vi "f_8_Tdoff.vi"(0 "file path (IN)":path, 1 "Project #":string, 2 "Request #":string, 3 "TEST #":string, 5 "error in (no error)":errorcluster, 6 "VGE":dbl, 8 "VCE":dbl) -> (14 "file path (OUT)":path, 15 "Tdoff (ns)":dbl, 16 "DONE Tdoff":bool, 19 "error out":errorcluster)   [LabVIEW 2020]
uses:
  GlobIndSw1.vi
  <vilib>/Waveform/WDTOps.llb/WDT Waveform Duration DBL.vi
  <vilib>/Waveform/WDTOps.llb/WDT Get Waveform Subset DBL.vi
  <vilib>/measure/mamon.llb/Trigger Detection for 1 Channel.vi
  <vilib>/Analysis/NI_AALBase.lvlib
  <vilib>/measure/NI_MAPro.lvlib
panel:
  in  "Decision ?":bool
  out "Cursor a : Channel 2":dbl
  out "Cursor a : Channel 3":dbl
  out "10% Vce":dbl
  out "90% Vge":dbl
  out "Waveform Graph":waveform(dbl)[](graph)
  out "OFF Region":waveform(dbl)[](graph) caption="Tdoff (ns)"
  # "Tdoff: from 90% Vge to 10% Vce"
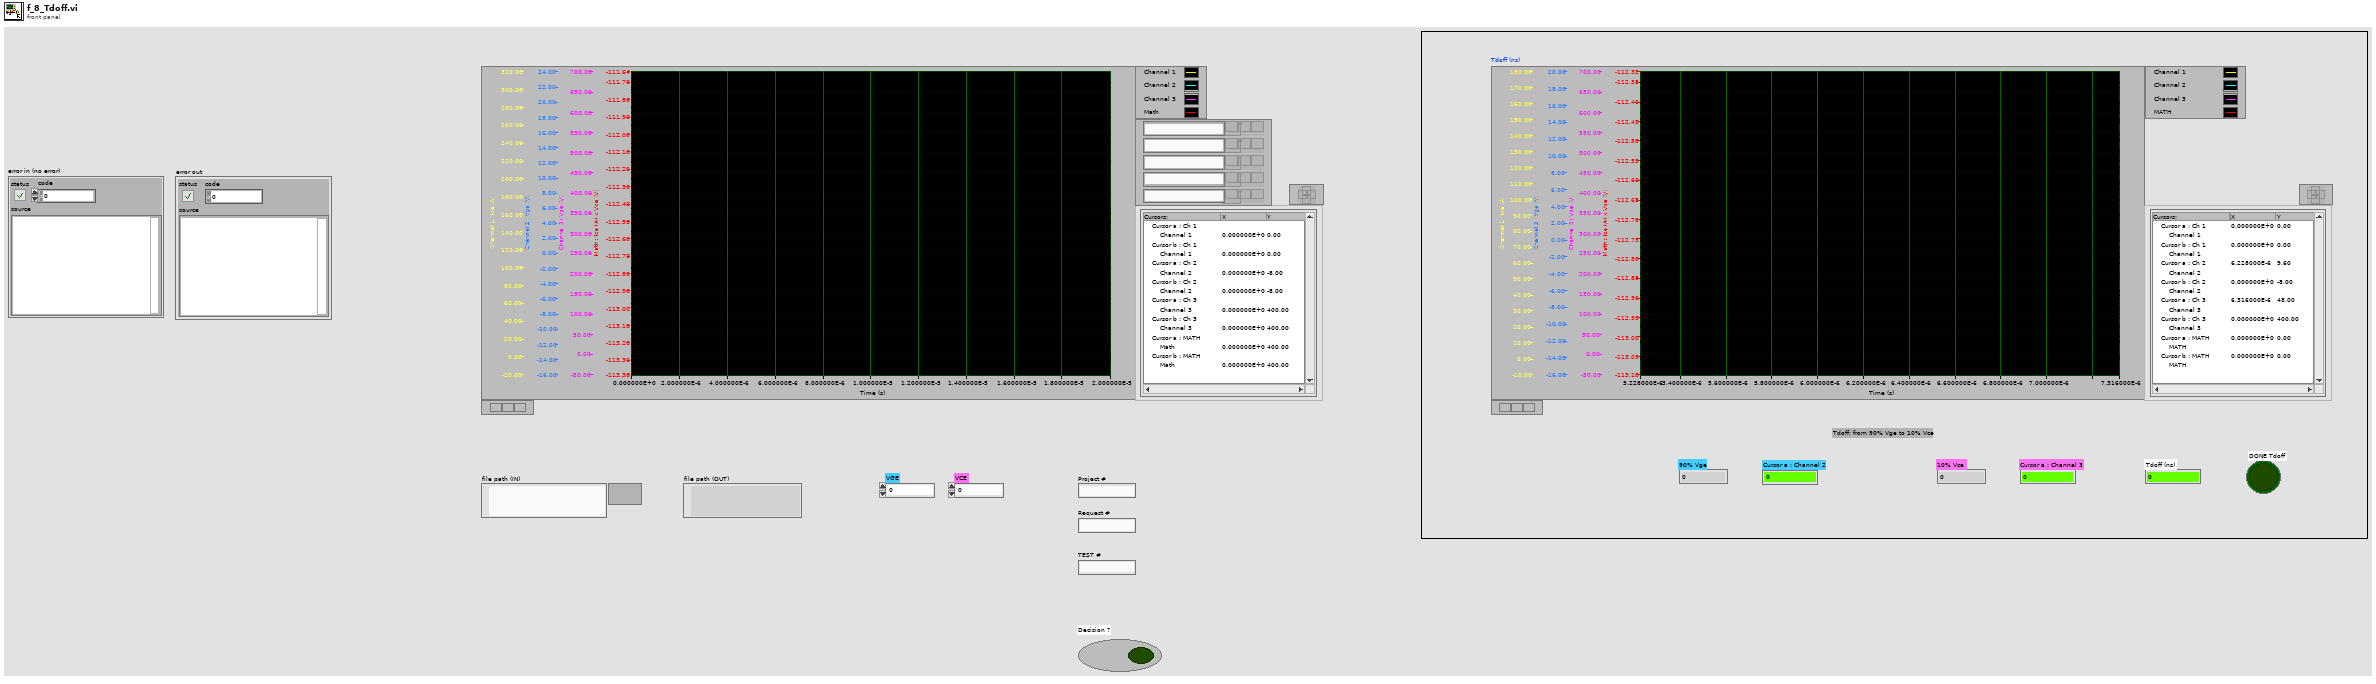
[diagram p1: front panel]
types:
  T1 = enum32{"Invalid", "Standard", "Closed", "Hidden", "Minimized", "Maximized"}
  T2 = typedef "imagedata.ctl" = cluster{"image type":i32, "image depth":i32, "image":u8[], "mask":u8[], "colors":u32[], "Rectangle":cluster{"left":i16, "top":i16, "right":i16, "bottom":i16}}
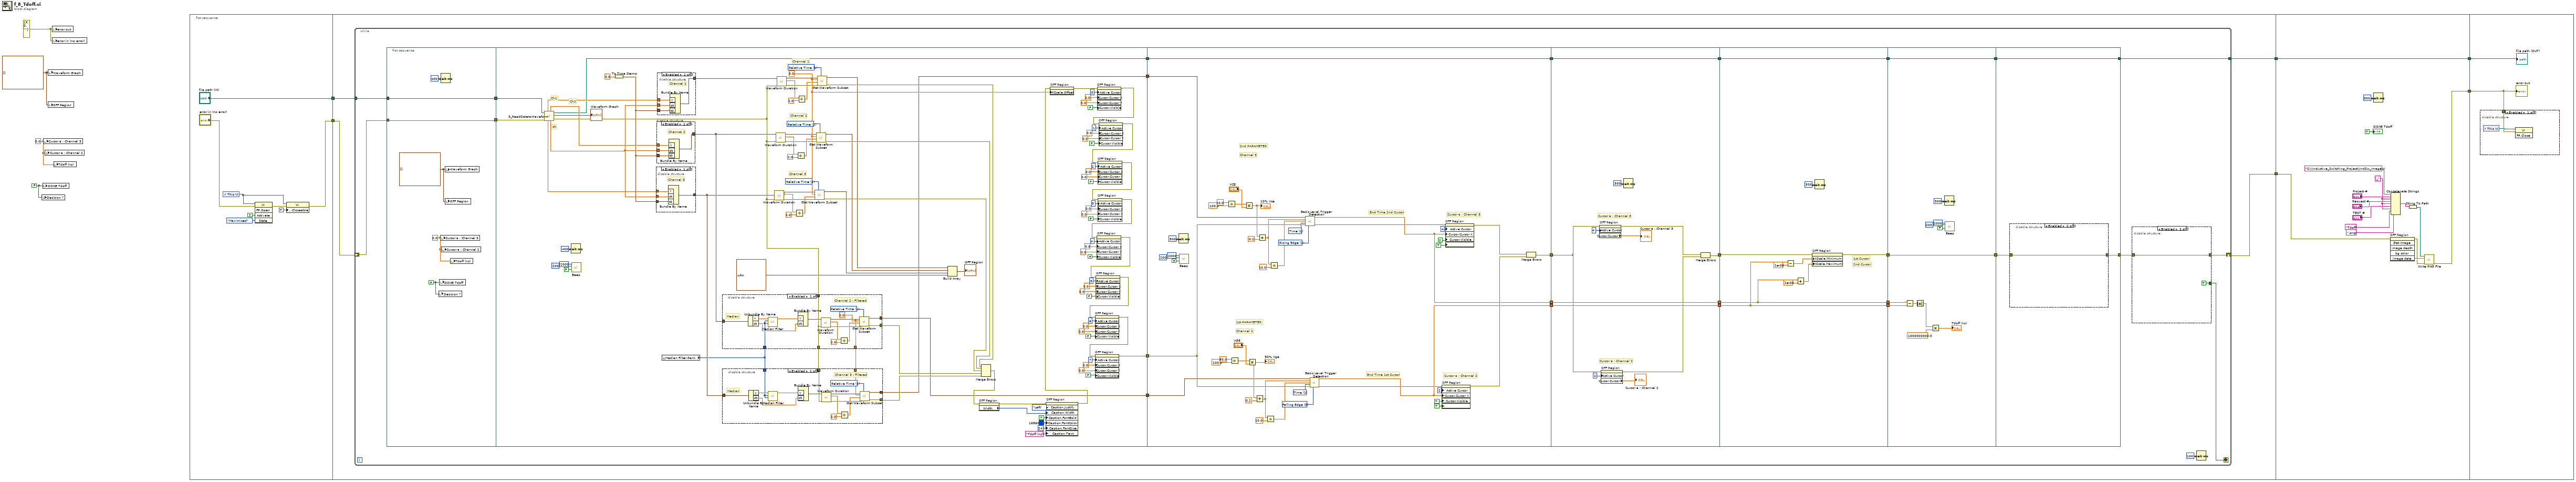
[diagram p0: block diagram]
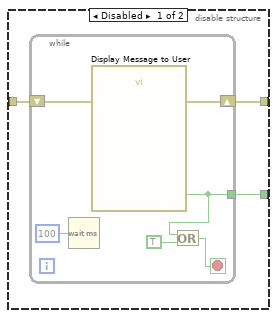
[diagram p2: hidden frame]
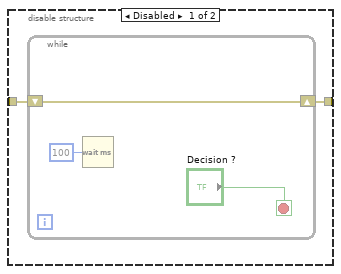
[diagram p8: hidden frame]
diagram:
  w2 = 0.0 ("Cursor a : Channel 3")
  w1 = FALSE ("DONE Tdon")
  w3 = waveform(dbl)[] [] ("Waveform Graph")
  w4 = errorcluster {"status"=FALSE, "code"=0, "source"=""} ("error out")
  n1 = local write "Decision ?"(w1) -> ()
  n2 = local write "DONE Tdoff"(w1) -> ()
  n3 = local write "Cursor a : Channel 3"(w2) -> ()
  n4 = local write "Cursor a : Channel 2"(w2) -> ()
  n5 = local write "Waveform Graph"(w3) -> ()
  n6 = local write "OFF Region"(w3) -> ()
  n7 = local write "error out"(w4) -> ()
  n8 = local write "error in (no error)"(w4) -> ()
  n9 = local write "Tdoff (ns)"(w2) -> ()
  n10 = flat-sequence {
    tunnel: ["file path (IN)"] -> w10
    tunnel: [w11] -> w9
    tunnel: w10 -> [w22]
    tunnel: [w21] -> w8
    tunnel: [w20] -> w7
    tunnel: w9 -> [w19]
    tunnel: w8 -> [w302]
    tunnel: w7 -> [w301]
    tunnel: [w301] -> w6
    tunnel: [w300] -> w5
    tunnel: w6 -> [w316]
    tunnel: w5 -> [w315]
    frame #0 {
      n11 = control-ref of="This VI"() -> (w16:refnum<vi>)
      n12 = invoke class="VI" method="FP.Open"(reference=w16, error in="error in (no error)", "Activate"=TRUE ("Activate?"), "State"=T1."Maximized") -> (error out=w17:errorcluster)  [unwired: 1 in, 4 out]
      n13 = property class="VI"(reference=w16, error in=w17, "Front Panel.Closeable"=TRUE ("Front Panel Window:Closeable")) -> (error out=w11:errorcluster)  [unwired: 1 out]
    }
    frame #1 {
      n14 = while {
        shift-right: [w27] -> w21
        shift-left: w19 -> [w23]
        tunnel: w22 -> [w25]
        tunnel: [w24] -> w20
        stop <- w28 stop-if-true
        n15 = flat-sequence {
          tunnel: [w62] -> w49
          tunnel: [w63] -> w48
          tunnel: w25 -> [w63]
          tunnel: w23 -> [w62]
          tunnel: w49 -> [w168]
          tunnel: w48 -> [w162]
          tunnel: [w71] -> w47
          tunnel: [w70] -> w46
          tunnel: [w92] -> w45
          tunnel: [w82] -> w44
          tunnel: w47 -> [w223]
          tunnel: w46 -> [w230]
          tunnel: w45 -> [w222]
          tunnel: [w229] -> w43
          tunnel: [w221] -> w42
          tunnel: [w238] -> w41
          tunnel: w44 -> [w237]
          tunnel: [w237] -> w40
          tunnel: w43 -> [w267]
          tunnel: [w267] -> w39
          tunnel: w42 -> [w266]
          tunnel: [w266] -> w38
          tunnel: w41 -> [w260]
          tunnel: [w257] -> w37
          tunnel: w40 -> [w265]
          tunnel: [w265] -> w36
          tunnel: w39 -> [w269]
          tunnel: [w269] -> w35
          tunnel: w38 -> [w270]
          tunnel: [w270] -> w34
          tunnel: w37 -> [w276]
          tunnel: [w275] -> w33
          tunnel: w36 -> [w277]
          tunnel: [w277] -> w32
          tunnel: w35 -> [w288]
          tunnel: w34 -> [w287]
          tunnel: w33 -> [w279]
          tunnel: w32 -> [w282]
          tunnel: [w282] -> w31
          tunnel: [w279] -> w30
          tunnel: w31 -> [w290]
          tunnel: w30 -> [w292]
          tunnel: [w291] -> w29
          tunnel: [w290] -> w24
          frame #0 {
            w65 = 0.0 ("Cursor a : Channel 3")
            w66 = FALSE ("DONE Tdon")
            w64 = waveform(dbl)[] [] ("Waveform Graph")
            n16 = local write "Decision ?"(w66) -> ()
            n17 = local write "DONE Tdoff"(w66) -> ()
            n18 = local write "Cursor a : Channel 3"(w65) -> ()
            n19 = Wait (ms)(milliseconds to wait=u32 400) -> ()  [unwired: 1 out]
            n20 = local write "Cursor a : Channel 2"(w65) -> ()
            n21 = local write "Waveform Graph"(w64) -> ()
            n22 = local write "OFF Region"(w64) -> ()
            n23 = local write "Tdoff (ns)"(w65) -> ()
          }
          frame #1 {
            w80 = 0.0 ("start samples/time")
            w143 = u16 1 items=["Samples", "Relative Time"] ("start/duration format")
            w154 = u16 1 items=["Samples", "Relative Time"] ("start/duration format")
            w155 = u16 1 items=["Samples", "Relative Time"] ("start/duration format")
            # "Channel 1"
            # "Channel 3"
            # "Channel 2"
            # "dt"
            # "Ch2"
            # "Ch1"
            n24 = call "3_ReadDatatoWaveform.vi"("error in (no error)"=w168, "file path (IN)"=w162) -> ("error out"=w75:errorcluster, "Waveform Graph"=→"Waveform Graph":waveform(dbl)[], "file path (OUT)"=w82:path, "dt"=w163:dbl, "Ch 2 Data"=w160:dbl[], "Ch 3 Data"=w164:dbl[], "Ch 1 Data"=w161:dbl[])  [unwired: 3 in]
            n25 = Wait (ms)(milliseconds to wait=u32 400) -> ()  [unwired: 1 out]
            n26 = call <vilib>:"Beep.vi"("use system alert? (T)"=FALSE, "duration (msec)"=u32 200, "frequency (Hz)"=u32 2000) -> ()  [unwired: 9 in]
            n27 = To Time Stamp(1:0.0 ("number")) -> (0:w165:timestamp)
            n28 = disable-structure shown="Enabled" {
              disable-tunnel: w165 -> [w212 _]
              disable-tunnel: w163 -> [w211 _]
              disable-tunnel: w164 -> [w210 _]
              disable-tunnel: [w209 _] -> w76
              frame Enabled {
                # "Channel 3"
                n29 = Bundle By Name("Y"=w210, "dt"=w211, "t0"=w212) -> (w209:waveform(dbl))  [unwired: 1 in]
              }
              frame Disabled {
              }
            }
            n30 = disable-structure shown="Enabled" {
              disable-tunnel: w165 -> [w208 _]
              disable-tunnel: w163 -> [w207 _]
              disable-tunnel: w160 -> [w206 _]
              disable-tunnel: [w205 _] -> w77
              frame Enabled {
                # "Channel 2"
                n31 = Bundle By Name("Y"=w206, "dt"=w207, "t0"=w208) -> (w205:waveform(dbl))  [unwired: 1 in]
              }
              frame Disabled {
              }
            }
            n32 = disable-structure shown="Enabled" {
              disable-tunnel: w165 -> [w204 _]
              disable-tunnel: w163 -> [w203 _]
              disable-tunnel: w161 -> [w202 _]
              disable-tunnel: [w201 _] -> w142
              frame Enabled {
                # "Channel 1"
                n33 = Bundle By Name("Y"=w202, "dt"=w203, "t0"=w204) -> (w201:waveform(dbl))  [unwired: 1 in]
              }
              frame Disabled {
              }
            }
            n34 = global read "GlobIndSw1.vi" "Median Filter Rank"() -> (w68:i32)
            n35 = disable-structure shown="Enabled" {
              disable-tunnel: w77 -> [w197 _]
              disable-tunnel: w75 -> [w187 _]
              disable-tunnel: [w189 _] -> w73
              disable-tunnel: [w188 _] -> w71
              disable-tunnel: [w187 _] -> w74
              disable-tunnel: [w186 _] -> w69
              disable-tunnel: w68 -> [w185 _]
              frame Enabled {
                w186 = 0.0 ("start samples/time")
                w191 = u16 1 items=["Samples", "Relative Time"] ("start/duration format")
                # "Channel 2 - Filtered"
                # "Median"
                n36 = Unbundle By Name(w197) -> ("Y"=w200:dbl[], "dt"=w198:dbl)
                n37 = call <vilib>:"Median Filter.vi"("right rank"=w185, "left rank"=w185, "X"=w200) -> ("Filtered X"=w199:dbl[])  [unwired: 7 in, 1 out]
                n38 = Bundle By Name("Y"=w199, "dt"=w198) -> (w190:waveform(dbl))  [unwired: 1 in]
                n39 = call-poly <vilib>:"Waveform Duration.vi"("error in (no error)"=w187, "waveform in"=w190) -> ("error out"=w194:errorcluster, "duration"=w196:dbl, "waveform out"=w195:waveform(dbl))  [unwired: 7 in]
                n40 = Divide(x=w196, y=2.0) -> (x/y=w193:dbl)
                n41 = call-poly <vilib>:"Get Waveform Subset.vi"("start/duration format"=w191, "error in (no error)"=w194, "duration"=w193, "start samples/time"=w186, "waveform in"=w195) -> ("error out"=w189:errorcluster, "waveform out"=w188:waveform(dbl))  [unwired: 1 in, 2 out]
              }
              frame Disabled {
              }
            }
            n42 = disable-structure shown="Enabled" {
              disable-tunnel: w76 -> [w181 _]
              disable-tunnel: w74 -> [w173 _]
              disable-tunnel: [w172 _] -> w72
              disable-tunnel: [w171 _] -> w70
              disable-tunnel: w69 -> [w170 _]
              disable-tunnel: w68 -> [w169 _]
              frame Enabled {
                w175 = u16 1 items=["Samples", "Relative Time"] ("start/duration format")
                # "Channel 3 - Filtered"
                # "Median"
                n43 = Unbundle By Name(w181) -> ("Y"=w184:dbl[], "dt"=w182:dbl)
                n44 = call <vilib>:"Median Filter.vi"("right rank"=w169, "left rank"=w169, "X"=w184) -> ("Filtered X"=w183:dbl[])  [unwired: 7 in, 1 out]
                n45 = Bundle By Name("Y"=w183, "dt"=w182) -> (w174:waveform(dbl))  [unwired: 1 in]
                n46 = call-poly <vilib>:"Waveform Duration.vi"("error in (no error)"=w173, "waveform in"=w174) -> ("error out"=w178:errorcluster, "duration"=w180:dbl, "waveform out"=w179:waveform(dbl))  [unwired: 7 in]
                n47 = Divide(x=w180, y=2.0) -> (x/y=w177:dbl)
                n48 = call-poly <vilib>:"Get Waveform Subset.vi"("start/duration format"=w175, "error in (no error)"=w178, "duration"=w177, "start samples/time"=w170, "waveform in"=w179) -> ("error out"=w172:errorcluster, "waveform out"=w171:waveform(dbl))  [unwired: 1 in, 2 out]
              }
              frame Disabled {
              }
            }
            n49 = call-poly <vilib>:"Waveform Duration.vi"("error in (no error)"=w75, "waveform in"=w76) -> ("error out"=w148:errorcluster, "duration"=w145:dbl, "waveform out"=w147:waveform(dbl))  [unwired: 7 in]
            n50 = call-poly <vilib>:"Waveform Duration.vi"("error in (no error)"=w75, "waveform in"=w77) -> ("error out"=w149:errorcluster, "duration"=w152:dbl, "waveform out"=w150:waveform(dbl))  [unwired: 7 in]
            n51 = call-poly <vilib>:"Waveform Duration.vi"("error in (no error)"=w75, "waveform in"=w142) -> ("error out"=w159:errorcluster, "duration"=w156:dbl, "waveform out"=w158:waveform(dbl))  [unwired: 7 in]
            n52 = Divide(x=w145, y=2.0) -> (x/y=w144:dbl)
            n53 = Divide(x=w152, y=2.0) -> (x/y=w153:dbl)
            n54 = Divide(x=w156, y=2.0) -> (x/y=w140:dbl)
            n55 = call-poly <vilib>:"Get Waveform Subset.vi"("start/duration format"=w143, "error in (no error)"=w148, "duration"=w144, "start samples/time"=w80, "waveform in"=w147) -> ("error out"=w79:errorcluster, "waveform out"=w81:waveform(dbl))  [unwired: 1 in, 2 out]
            n56 = call-poly <vilib>:"Get Waveform Subset.vi"("start/duration format"=w154, "error in (no error)"=w149, "duration"=w153, "start samples/time"=w80, "waveform in"=w150) -> ("error out"=w138:errorcluster, "waveform out"=w94:waveform(dbl))  [unwired: 1 in, 2 out]
            n57 = call-poly <vilib>:"Get Waveform Subset.vi"("start/duration format"=w155, "error in (no error)"=w159, "duration"=w140, "start samples/time"=w80, "waveform in"=w158) -> ("error out"=w139:errorcluster, "waveform out"=w93:waveform(dbl))  [unwired: 1 in, 2 out]
            n58 = Build Array(w93, w94, w81, waveform(dbl) {"t0"=timestamp(0 s since 1904-01-01), "dt"=1.0, "Y"=[]} ("element")) -> (→"OFF Region":waveform(dbl)[])
            n59 = Merge Errors(w139, w138, w79, w73, w72) -> (w90:errorcluster)
            n60 = property on="OFF Region" class="WFGraph (strict)"(error in=w90) -> (error out=w89:errorcluster, "Width"=w88:u32)  [unwired: 1 in, 1 out]
            n61 = property on="OFF Region" class="WFGraph (strict)"(error in=w89, "Caption.Justify"=enum16{"Left", "Center", "Right"}."Left" ("Caption.Justification"), "Caption.Width"=w88, "Caption.FontBold"=TRUE ("Caption.Font:Bold"), "Caption.FontColor"=u32 16860 ("Caption.Font:Color"), "Caption.FontSize"=u32 24 ("Caption.Font:Size"), "Caption.Text"="Tdoff (ns)") -> (error out=w84:errorcluster)  [unwired: 1 in, 1 out]
            n62 = property on="OFF Region" class="WFGraph (strict)"(error in=w84, "XScale.Offset"=w80) -> (error out=w118:errorcluster)  [unwired: 1 in, 1 out]
            n63 = property on="OFF Region" class="WFGraph (strict)"(error in=w118, "Active Cursor"=u32 0, "Cursor.Cursor X"=0.0 ("Cursor.Cursor Position:Cursor X"), "Cursor.Cursor Y"=0.0 ("Cursor.Cursor Position:Cursor Y"), "Cursor.Visible"=FALSE) -> (error out=w117:errorcluster)  [unwired: 1 in, 1 out]
            n64 = property on="OFF Region" class="WFGraph (strict)"(error in=w117, "Active Cursor"=u32 1, "Cursor.Cursor X"=0.0 ("Cursor.Cursor Position:Cursor X"), "Cursor.Cursor Y"=0.0 ("Cursor.Cursor Position:Cursor Y"), "Cursor.Visible"=FALSE) -> (error out=w116:errorcluster)  [unwired: 1 in, 1 out]
            n65 = property on="OFF Region" class="WFGraph (strict)"(error in=w116, "Active Cursor"=u32 2, "Cursor.Cursor X"=0.0 ("Cursor.Cursor Position:Cursor X"), "Cursor.Cursor Y"=0.0 ("Cursor.Cursor Position:Cursor Y"), "Cursor.Visible"=FALSE) -> (error out=w115:errorcluster)  [unwired: 1 in, 1 out]
            n66 = property on="OFF Region" class="WFGraph (strict)"(error in=w115, "Active Cursor"=u32 3, "Cursor.Cursor X"=0.0 ("Cursor.Cursor Position:Cursor X"), "Cursor.Cursor Y"=0.0 ("Cursor.Cursor Position:Cursor Y"), "Cursor.Visible"=FALSE) -> (error out=w98:errorcluster)  [unwired: 1 in, 1 out]
            n67 = property on="OFF Region" class="WFGraph (strict)"(error in=w98, "Active Cursor"=u32 4, "Cursor.Cursor X"=0.0 ("Cursor.Cursor Position:Cursor X"), "Cursor.Cursor Y"=0.0 ("Cursor.Cursor Position:Cursor Y"), "Cursor.Visible"=FALSE) -> (error out=w97:errorcluster)  [unwired: 1 in, 1 out]
            n68 = property on="OFF Region" class="WFGraph (strict)"(error in=w97, "Active Cursor"=u32 5, "Cursor.Cursor X"=0.0 ("Cursor.Cursor Position:Cursor X"), "Cursor.Cursor Y"=0.0 ("Cursor.Cursor Position:Cursor Y"), "Cursor.Visible"=FALSE) -> (error out=w96:errorcluster)  [unwired: 1 in, 1 out]
            n69 = property on="OFF Region" class="WFGraph (strict)"(error in=w96, "Active Cursor"=u32 6, "Cursor.Cursor X"=0.0 ("Cursor.Cursor Position:Cursor X"), "Cursor.Cursor Y"=0.0 ("Cursor.Cursor Position:Cursor Y"), "Cursor.Visible"=FALSE) -> (error out=w95:errorcluster)  [unwired: 1 in, 1 out]
            n70 = property on="OFF Region" class="WFGraph (strict)"(error in=w95, "Active Cursor"=u32 7, "Cursor.Cursor X"=0.0 ("Cursor.Cursor Position:Cursor X"), "Cursor.Cursor Y"=0.0 ("Cursor.Cursor Position:Cursor Y"), "Cursor.Visible"=FALSE) -> (error out=w92:errorcluster)  [unwired: 1 in, 1 out]
          }
          frame #2 {
            w226 = u16 0 items=["Falling Edge", "Rising Edge"] ("trigger slope")
            w227 = u16 1 items=["Index", "Time"] ("location mode")
            w233 = u16 1 items=["Falling Edge", "Rising Edge"] ("trigger slope")
            w234 = u16 1 items=["Index", "Time"] ("location mode")
            # "Cursor a : Channel 2"
            # "Cursor a : Channel 3"
            # "End Time 2nd Cursor"
            # "End Time 1st Cursor"
            # "2nd PARAMETER"
            # "Channel 3"
            # "1st PARAMETER"
            # "Channel 2"
            n71 = Wait (ms)(milliseconds to wait=u32 500) -> ()  [unwired: 1 out]
            n72 = call <vilib>:"Beep.vi"("use system alert? (T)"=FALSE, "duration (msec)"=u32 200, "frequency (Hz)"=u32 2000) -> ()  [unwired: 9 in]
            n73 = Divide(x=10.0, y=100.0) -> (x/y=w255:dbl)
            n74 = Divide(x=90.0, y=100.0) -> (x/y=w251:dbl)
            n75 = Multiply(x=w255, y="VCE") -> (x*y=w231:dbl)
            "10% Vce" <- w231
            n76 = Multiply(x=w251, y="VGE") -> (x*y=w224:dbl)
            "90% Vge" <- w224
            n77 = Add(x=w224, y=0.2) -> (x+y=w218:dbl)
            n78 = Add(x=w231, y=0.2) -> (x+y=w215:dbl)
            n79 = Divide(x=w218, y=10.0) -> (x/y=w217:dbl)
            n80 = Divide(x=w215, y=10.0) -> (x/y=w214:dbl)
            n81 = call-poly <vilib>:"Basic Level Trigger Detection.vi"("signal in"=w230, "level"=w215, "hysteresis"=w214, "location mode"=w234, "error in (no error)"=w222, "trigger slope"=w233) -> ("trigger location"=w229:dbl, "error out"=w228:errorcluster)  [unwired: 7 in, 1 out]
            n82 = call-poly <vilib>:"Basic Level Trigger Detection.vi"("signal in"=w223, "level"=w218, "hysteresis"=w217, "location mode"=w227, "error in (no error)"=w222, "trigger slope"=w226) -> ("trigger location"=w221:dbl, "error out"=w220:errorcluster)  [unwired: 7 in, 1 out]
            n83 = property on="OFF Region" class="WFGraph (strict)"(error in=w220, "Active Cursor"=u32 2, "Cursor.Cursor X"=w221, "Cursor.Visible"=TRUE, "Cursor.Cursor Name Visible"=TRUE) -> (error out=w239:errorcluster)  [unwired: 1 in, 1 out]
            n84 = property on="OFF Region" class="WFGraph (strict)"(error in=w228, "Active Cursor"=u32 4, "Cursor.Cursor X"=w229, "Cursor.Visible"=TRUE, "Cursor.Cursor Name Visible"=TRUE) -> (error out=w240:errorcluster)  [unwired: 1 in, 1 out]
            n85 = Merge Errors(w240, w239) -> (w238:errorcluster)
          }
          frame #3 {
            # "Cursor a : Channel 3"
            # "Cursor a : Channel 2"
            n86 = property on="OFF Region" class="WFGraph (strict)"(error in=w260, "Active Cursor"=u32 4) -> (error out=w259:errorcluster, "Cursor.Cursor Y"=→"Cursor a : Channel 3":dbl)  [unwired: 1 in, 1 out]
            n87 = property on="OFF Region" class="WFGraph (strict)"(error in=w260, "Active Cursor"=u32 2) -> (error out=w258:errorcluster, "Cursor.Cursor Y"=→"Cursor a : Channel 2":dbl)  [unwired: 1 in, 1 out]
            n88 = Wait (ms)(milliseconds to wait=u32 300) -> ()  [unwired: 1 out]
            n89 = Merge Errors(w259, w258) -> (w257:errorcluster)
          }
          frame #4 {
            # "2nd Cursor"
            # "1st Cursor"
            n90 = Subtract(x=w270, y=1e-06) -> (x-y=w271:dbl)
            n91 = Add(x=w269, y=1e-06) -> (x+y=w272:dbl)
            n92 = property on="OFF Region" class="WFGraph (strict)"(error in=w276, "XScale.Minimum"=w271, "XScale.Maximum"=w272) -> (error out=w275:errorcluster)  [unwired: 1 in, 1 out]
            n93 = Wait (ms)(milliseconds to wait=u32 300) -> ()  [unwired: 1 out]
          }
          frame #5 {
            n94 = Subtract(x=w288, y=w287) -> (x-y=w281:dbl)
            n95 = Absolute Value(x=w281) -> (abs(x)=w280:dbl)
            n96 = Multiply(x=w280, y=1000000000.0) -> (x*y=→"Tdoff (ns)":dbl)
            n97 = Wait (ms)(milliseconds to wait=u32 300) -> ()  [unwired: 1 out]
            n98 = call <vilib>:"Beep.vi"("use system alert? (T)"=FALSE, "duration (msec)"=u32 200, "frequency (Hz)"=u32 2000) -> ()  [unwired: 9 in]
          }
          frame #6 {
            n99 = disable-structure shown="Enabled" {
              disable-tunnel: w292 -> [w294 w298]
              disable-tunnel: [w293 w298] -> w291
              frame Disabled {
                n100 = while {
                  shift-right: [w295] -> w293
                  shift-left: w294 -> [w295]
                  stop <- "Decision ?" stop-if-true
                  n101 = Wait (ms)(milliseconds to wait=u32 100) -> ()  [unwired: 1 out]
                }
              }
              frame Enabled {
              }
            }
          }
        }
        n102 = disable-structure shown="Enabled" {
          disable-tunnel: w29 -> [w52 w60]
          disable-tunnel: [w51 TRUE ("NO")] -> w28
          disable-tunnel: [w50 w60] -> w27
          frame Disabled {
            n103 = while {
              tunnel: [w54] -> w51
              shift-right: [w57] -> w50
              shift-left: w52 -> [w58]
              stop <- w56 stop-if-true
              n104 = Wait (ms)(milliseconds to wait=u32 100) -> ()  [unwired: 1 out]
              n105 = call "Display Message to User"("error in (no error)"=w58) -> ("error out"=w57:errorcluster, "NO"=w54:bool)  [unwired: 9 in]
              n106 = Or(x=w54, y=TRUE) -> (x .or. y?=w56:bool)
            }
          }
          frame Enabled {
          }
        }
        n107 = Wait (ms)(milliseconds to wait=u32 100) -> ()  [unwired: 1 out]
      }
    }
    frame #2 {
      w306 = "_"
      n108 = Wait (ms)(milliseconds to wait=u32 300) -> ()  [unwired: 1 out]
      n109 = invoke on="OFF Region" class="WFGraph (strict)" method="Get Image"(error in=w302) -> (error out=w308:errorcluster, "image data"=w311:T2)  [unwired: 5 in, 4 out]
      n110 = Concatenate Strings("C:\\Inductive_Switching_Project\\IndSw_Image\\" ("string"), "Project #", w306, "Request #", w306, "TEST #", w306, "Tdoff" ("string"), ".png" ("string")) -> (w312:string)
      n111 = String To Path(string=w312) -> (path=w310:path)
      n112 = call <vilib>:"Write PNG File.vi"("error in (no error)"=w308, "image data"=w311, "path to PNG file"=w310) -> ("error out"=w300:errorcluster)  [unwired: 7 in, 1 out]
      "DONE Tdoff" <- TRUE ("DONE Tdon")
    }
    frame #3 {
      n113 = disable-structure shown="Enabled" {
        disable-tunnel: w315 -> [w317 _]
        frame Enabled {
          n114 = control-ref of="This VI"() -> (w318:refnum<vi>)
          n115 = invoke class="VI" method="FP.Close"(reference=w318, error in=w317) -> ()  [unwired: 1 in, 3 out]
        }
        frame Disabled {
        }
      }
      "error out" <- w315
      "file path (OUT)" <- w316
    }
  }
